vi "Read Write.vi"() -> ()   [LabVIEW 2020]
uses:
  1f30cec2-9676-4920-9d1c-916661d95807.vi
  1f30cec2-9676-4920-9d1c-916661d95807.vi/0a801874-4294-4bdb-9e47-e4688f1d83ac.vi
  1f30cec2-9676-4920-9d1c-916661d95807.vi/6cca9ae9-92c3-46a2-9678-29acf2e71fda.vi
  1f30cec2-9676-4920-9d1c-916661d95807.vi/0a801874-4294-4bdb-9e47-e4688f1d83ac.vi/fb80aafa-2e1d-4838-8f30-9efae5849591.vi
  1f30cec2-9676-4920-9d1c-916661d95807.vi/0a801874-4294-4bdb-9e47-e4688f1d83ac.vi/8fdc059d-7f2d-4fa3-8c52-051ce8525472.vi
  1f30cec2-9676-4920-9d1c-916661d95807.vi/6cca9ae9-92c3-46a2-9678-29acf2e71fda.vi/b1633edd-83f7-4da2-9535-b0b292f027f0.vi
  1f30cec2-9676-4920-9d1c-916661d95807.vi/6cca9ae9-92c3-46a2-9678-29acf2e71fda.vi/6ba00d27-a418-4eed-9d93-56a1082e19cc.vi
  1f30cec2-9676-4920-9d1c-916661d95807.vi/0a801874-4294-4bdb-9e47-e4688f1d83ac.vi/8fdc059d-7f2d-4fa3-8c52-051ce8525472.vi/b1633edd-83f7-4da2-9535-b0b292f027f0.vi
  1f30cec2-9676-4920-9d1c-916661d95807.vi/0a801874-4294-4bdb-9e47-e4688f1d83ac.vi/8fdc059d-7f2d-4fa3-8c52-051ce8525472.vi/6ba00d27-a418-4eed-9d93-56a1082e19cc.vi
  Source/Classes/Pointer/Check Move.vi
  Source/Classes/Pointer/Is Error.vi
  Source/Classes/Pointer/Get Address.vi
  Source/Classes/Pointer/Write 1D DBL.vi
  Source/Classes/Pointer/Pointer.lvclass
panel:
  out "read error":errorcluster
  out "write error":errorcluster
  out "read buffer":dbl[](array[numeric])
  in  "write buffer":dbl[](array[numeric])
  in  "stop":bool
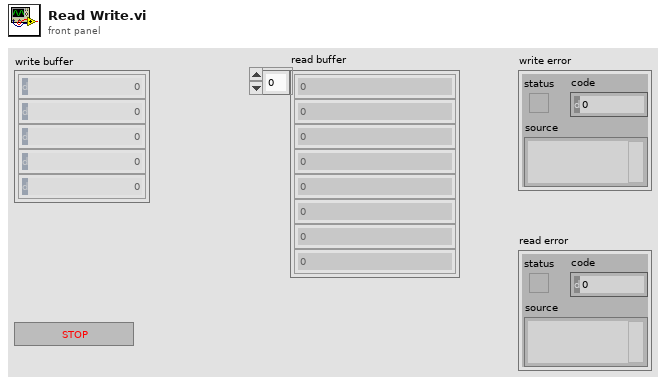
[diagram p1: front panel]
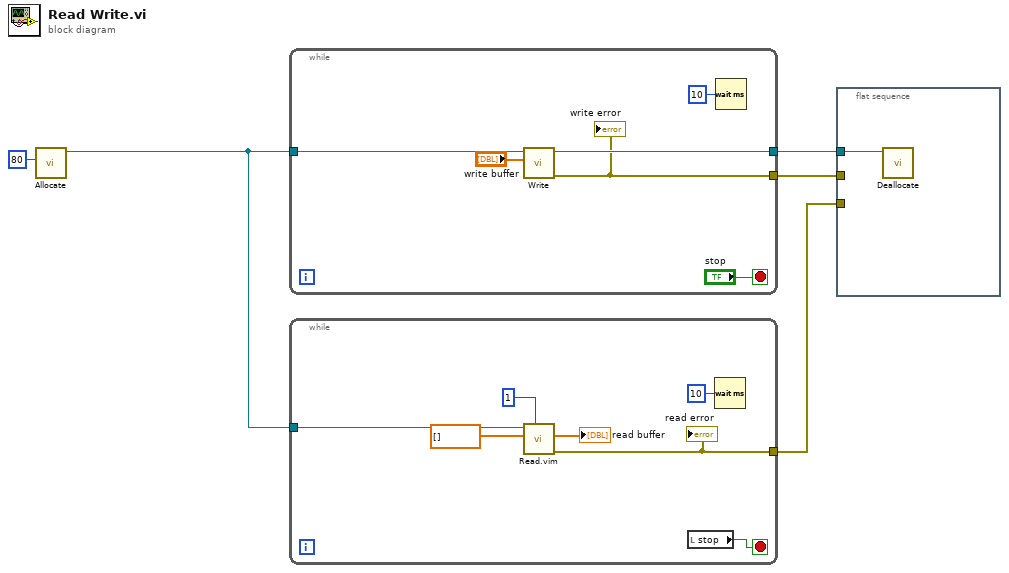
[diagram p0: block diagram]
diagram:
  n1 = call "Allocate.vi"("size"=u64 80) -> ("Pointer out"=w1:refnum<class "Pointer.lvclass">)  [unwired: 9 in, 1 out]
  n2 = while {
    tunnel: w1 -> [w11]
    tunnel: [w10] -> w4
    tunnel: [w9] -> w3
    stop <- "stop" stop-if-true
    n3 = call-poly "Write.vi"("buffer in"="write buffer", "Pointer in"=w11) -> ("error out"=w9:errorcluster, "Pointer out"=w10:refnum<class "Pointer.lvclass">)  [unwired: 6 in, 2 out]
    "write error" <- w9
    n4 = Wait (ms)(milliseconds to wait=u32 10) -> ()  [unwired: 1 out]
  }
  n5 = while {
    tunnel: [w18] -> w2
    tunnel: w1 -> [w15]
    stop <- w17 stop-if-true
    n6 = call "Read.vim"("count (-1: rest)"=i64 1, "buffer in"=dbl[] [], "Pointer in"=w15) -> ("error out"=w18:errorcluster, "buffer out"=→"read buffer":dbl[])  [unwired: 5 in, 2 out]
    "read error" <- w18
    n7 = local read "stop"() -> (w17:bool)
    n8 = Wait (ms)(milliseconds to wait=u32 10) -> ()  [unwired: 1 out]
  }
  n9 = flat-sequence {
    tunnel: w4 -> [w19]
    tunnel: w3 -> [_]
    tunnel: w2 -> [_]
    frame #0 {
      n10 = call "Deallocate.vi"("Pointer"=w19) -> ()  [unwired: 9 in, 2 out]
    }
  }
